vi "PrintConsole.vi"() -> ()   [LabVIEW 2013]
doc: "Vous devez créer un VI Console d’impression qui contrôle les soumissions\nde travaux d’impression et surveille l’état du traitement des travaux\nd’impression. Chaque fois que l’utilisateur clique sur le bouton Événement\nde file d’attente, un travail d’impression sera envoyé à l’imprimante. Vous\nsurveillerez le nombre de travaux d’impression dans la file d’attente en\nutilisant une barre verticale. Des LED indiqueront l’état du traitement de\nl’impression.\nLe processus d’impression pour chaque travail inclut deux étapes : une\nphase d’initialisation d’une durée fixe de 300 ms et une phase d’impression\ndont la durée varie en fonction de la taille du document à imprimer"
uses:
  Print LEDs.ctl
  Print Processing States.ctl
panel:
  out "nb d'éléments dans la file d'attente":i32
  in  "Evenement Fille Atente\nEvenement Fille Atente":bool
  in  "stop":bool
  out "LED d'impression":T1={"En attente"=TRUE, "Initialisation"=FALSE, "Impression"=FALSE}
  out "Travaux d'impression\nen file d'attente":i32(slide) scale=0.0..25.0
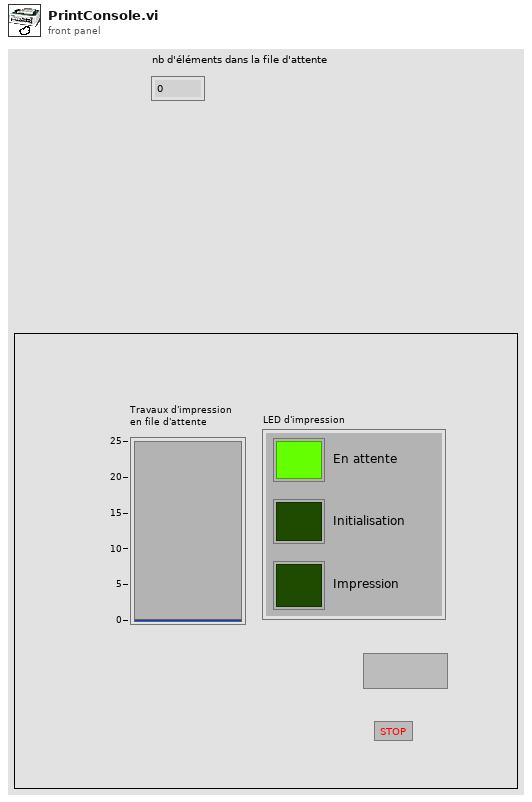
[diagram p1: front panel]
types:
  T1 = typedef "Print LEDs.ctl" = cluster{"En attente":bool, "Initialisation":bool, "Impression":bool}
  T2 = typedef "Print Processing States.ctl" = enum16{"En attente", "Initialisation de la configuration", "Configuration", "Initialisation de l'impression", "Impression"}
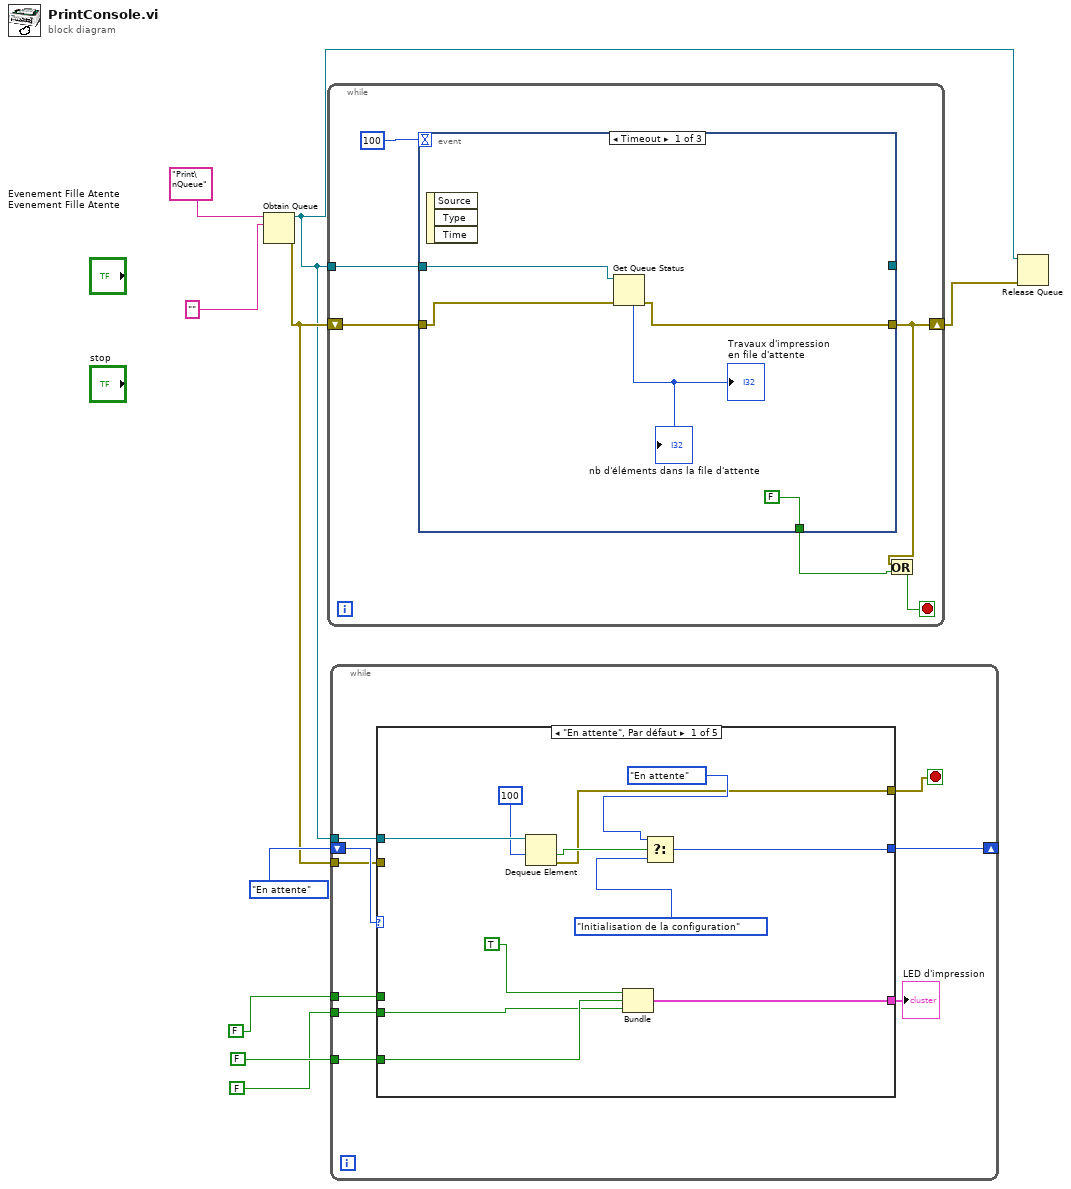
[diagram p0: block diagram]
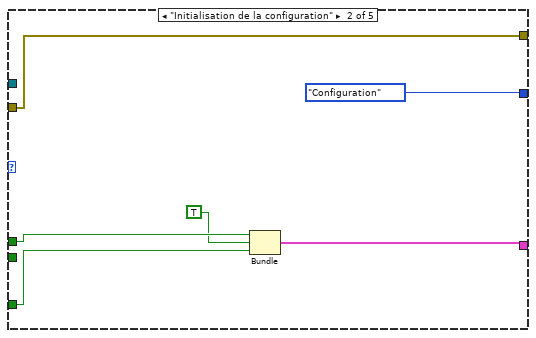
[diagram p2: hidden frame]
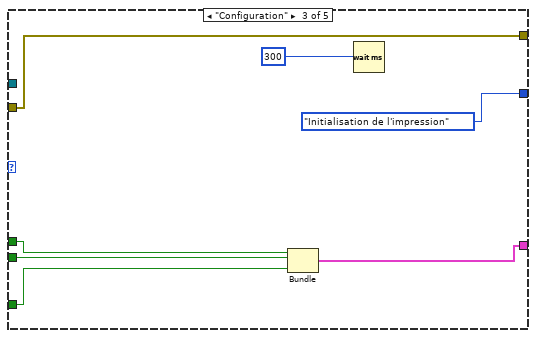
[diagram p3: hidden frame]
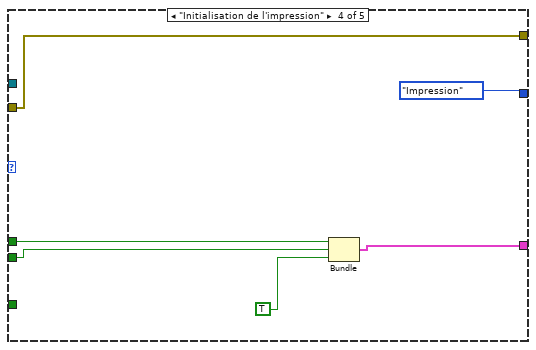
[diagram p4: hidden frame]
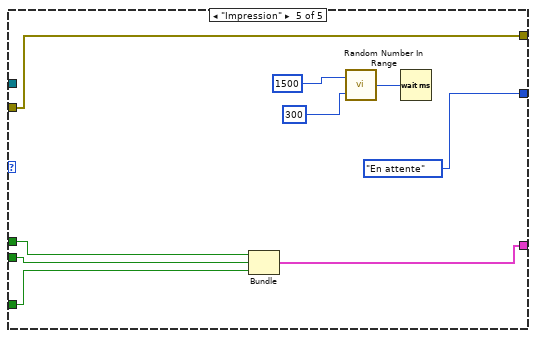
[diagram p5: hidden frame]
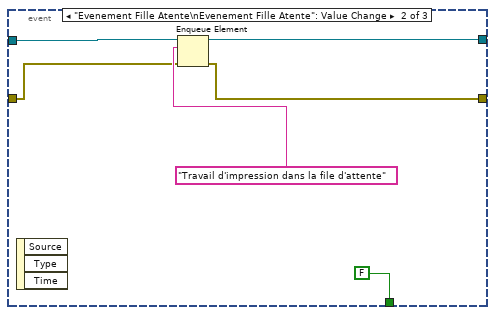
[diagram p6: hidden frame]
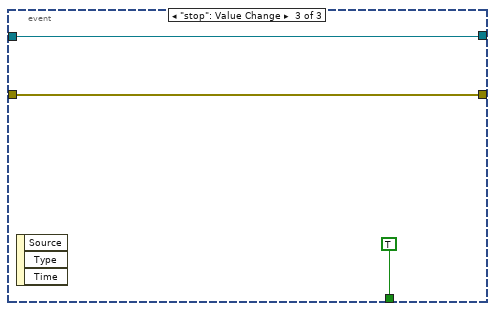
[diagram p7: hidden frame]
diagram:
  n1 = Obtain Queue(name (unnamed)="Print\nQueue", element data type="") -> (queue out=w4:refnum<queue>, error out=w5:errorcluster)  [unwired: 3 in, 1 out]
  n2 = while {
    tunnel: w4 -> [w15]
    shift-right: [w13] -> w7
    shift-left: w5 -> [w14]
    stop <- w11 stop-if-true
    n3 = event shown="[0] Timeout" {
      selector: _ -> [_ _ _]
      dyn-events: _ -> [_ _ _]
      timeout: 100 -> [_ _ _]
      tunnel: w15 -> [w16 w26 w28]
      tunnel: [_ w24 w28] -> _
      tunnel: [FALSE FALSE TRUE] -> w12
      tunnel: w14 -> [w18 w22 w27]
      tunnel: [w17 w21 w27] -> w13
      event Timeout {
        n4 = event-data() -> ()  [unwired: 1 in, 3 out]
        n5 = Get Queue Status(queue=w16, error in (no error)=w18) -> (error out=w17:errorcluster, # elements in queue=→"Travaux d'impression\nen file d'attente" →"nb d'éléments dans la file d'attente":i32)  [unwired: 1 in, 6 out]
      }
      event "Evenement Fille Atente\nEvenement Fille Atente": Value Change {
        n6 = event-data() -> ()  [unwired: 1 in, 3 out]
        n7 = Enqueue Element(queue=w26, element="Travail d'impression dans la file d'attente", error in (no error)=w22) -> (queue out=w24:refnum<queue>, error out=w21:errorcluster)  [unwired: 1 in, 1 out]
      }
      event "stop": Value Change {
        n8 = event-data() -> ()  [unwired: 1 in, 3 out]
      }
    }
    n9 = Or(x=w13, y=w12) -> (x .or. y?=w11:bool)
  }
  n10 = while {
    tunnel: w5 -> [w37]
    tunnel: w4 -> [w36]
    shift-right: [w35] -> _
    shift-left: Print_Processing_States."En attente" ("Énum") -> [w38]
    tunnel: FALSE -> [w34]
    tunnel: FALSE -> [w33]
    tunnel: FALSE -> [w32]
    stop <- w30 stop-if-true
    n11 = case shown="\"En attente\", Par défaut" w38 {
      tunnel: w37 -> [_ w50 w56 w63 w69]
      tunnel: w36 -> [w49 _ _ _ _]
      tunnel: [w44 Print_Processing_States."Configuration" ("Énum 2") Print_Processing_States."Initialisation de l'impression" ("Énum 2") Print_Processing_States."Impression" ("Énum 2") Print_Processing_States."En attente" ("Énum 2")] -> w35
      tunnel: w34 -> [_ w55 w61 w66 w72]
      tunnel: w33 -> [w43 w54 w59 _ w74]
      tunnel: w32 -> [w42 _ w60 w67 w73]
      tunnel: [w40 w52 w58 w65 w71] -> w31
      tunnel: [w39 w50 w56 w63 w69] -> w30
      frame "En attente", Default {
        n12 = Dequeue Element(queue=w49, timeout in ms (-1)=100) -> (timed out?=w47:bool, error out=w39:errorcluster)  [unwired: 1 in, 2 out]
        n13 = Bundle(TRUE, w43, w42) -> (w40:cluster{bool, bool, bool})  [unwired: 1 in]
        n14 = Select(t=Print_Processing_States."En attente" ("Énum 2"), s=w47, f=Print_Processing_States."Initialisation de la configuration" ("Énum 2")) -> (s? t:f=w44:T2)
      }
      frame "Initialisation de la configuration" {
        n15 = Bundle(w55, TRUE, w54) -> (w52:cluster{bool, bool, bool})  [unwired: 1 in]
      }
      frame "Configuration" {
        n16 = Bundle(w61, w60, w59) -> (w58:cluster{bool, bool, bool})  [unwired: 1 in]
        n17 = Wait (ms)(milliseconds to wait=300) -> ()  [unwired: 1 out]
      }
      frame "Initialisation de l'impression" {
        n18 = Bundle(w66, w67, TRUE) -> (w65:cluster{bool, bool, bool})  [unwired: 1 in]
      }
      frame "Impression" {
        n19 = Bundle(w72, w73, w74) -> (w71:cluster{bool, bool, bool})  [unwired: 1 in]
        n20 = call "Random Number In Range.vi"("Limite inférieure"=300, "Limite supérieure"=1500) -> ("Nb aléatoire"=w75:u32)
        n21 = Wait (ms)(milliseconds to wait=w75) -> ()  [unwired: 1 out]
      }
    }
    "LED d'impression" <- w31
  }
  n22 = Release Queue(queue=w4, error in (no error)=w7) -> ()  [unwired: 1 in, 3 out]
